vi "Patrycja_2.vi"() -> ()   [LabVIEW 2025]
uses:
  <vilib>/Instr/_visa.llb/VISA Flush IO Buffer Mask.ctl
  <vilib>/Utility/error.llb/Trim Whitespace One-Sided.vi
  <vilib>/Instr/_visa.llb/VISA Configure Serial Port (Instr).vi
panel:
  in  "Tab Control":T1(tab)
  out "Thermometer":dbl(slide) scale=0.0..100.0
  out "Temperatura wykres":dbl(graph)
  out "Temperatura liczba":dbl
  out "Temperatura max [C]":dbl
  out "Temperatura min[C]":dbl
  out "Temperatura średnia[C]":dbl
  out "Wilgotność wykres":dbl(graph)
  out "Tank":dbl(slide) scale=0.0..100.0
  out "wilgotność liczba":dbl
  out "Wilgotnosc max [%]":dbl
  out "Wilogtność min [%]":dbl
  out "Wilgotność średnia[%]":dbl
  out "Bardzo Suche":bool
  out "Punkt Rosy":dbl format="%#_4g"
  out "Indeks ciepła":dbl format="%#_4g"
  out "Suche":bool
  out "Komfort":bool
  out "Wilgotno":bool
  out "Bardzo Wilgotno":bool
  out "Komfort":bool
  out "Uwaga":bool
  out "Duża Ostrożność":bool
  out "Niebezpieczne":bool
  out "Ekstremalnie niebezpieczne":bool
  out "wyświetlanie danych":string
  out "Czy dziła whlie":i32
  out "numeric - start/stop":dbl
  in  "START/STOP":bool
  out "wyświetlanie danych 2":string
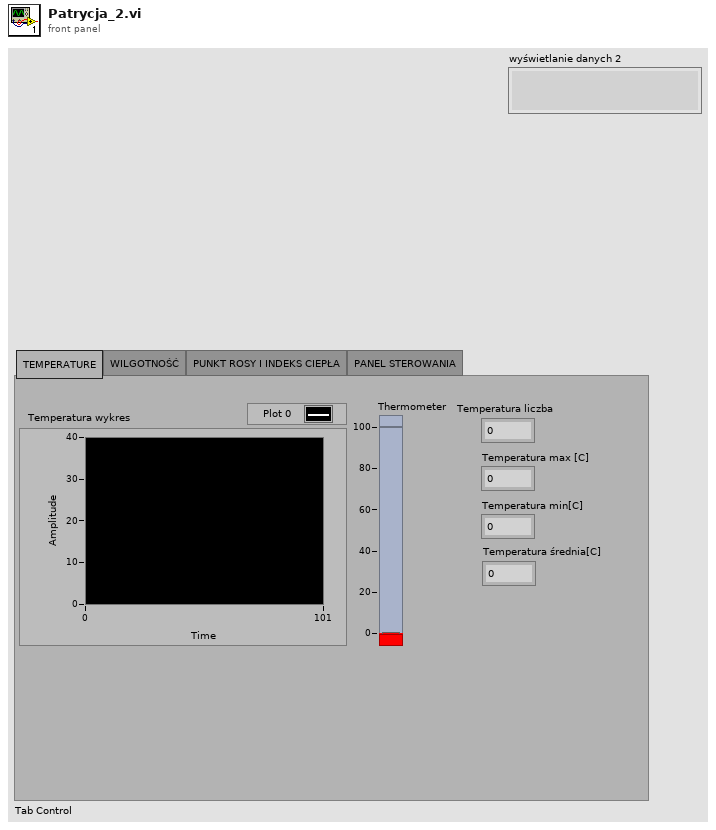
[diagram p1: front panel]
types:
  T1 = enum32{"TEMPERATURE", "WILGOTNOŚĆ", "PUNKT ROSY I INDEKS CIEPŁA", "PANEL STEROWANIA"}
  T2 = typedef "VISA Flush IO Buffer Mask.ctl" = u16
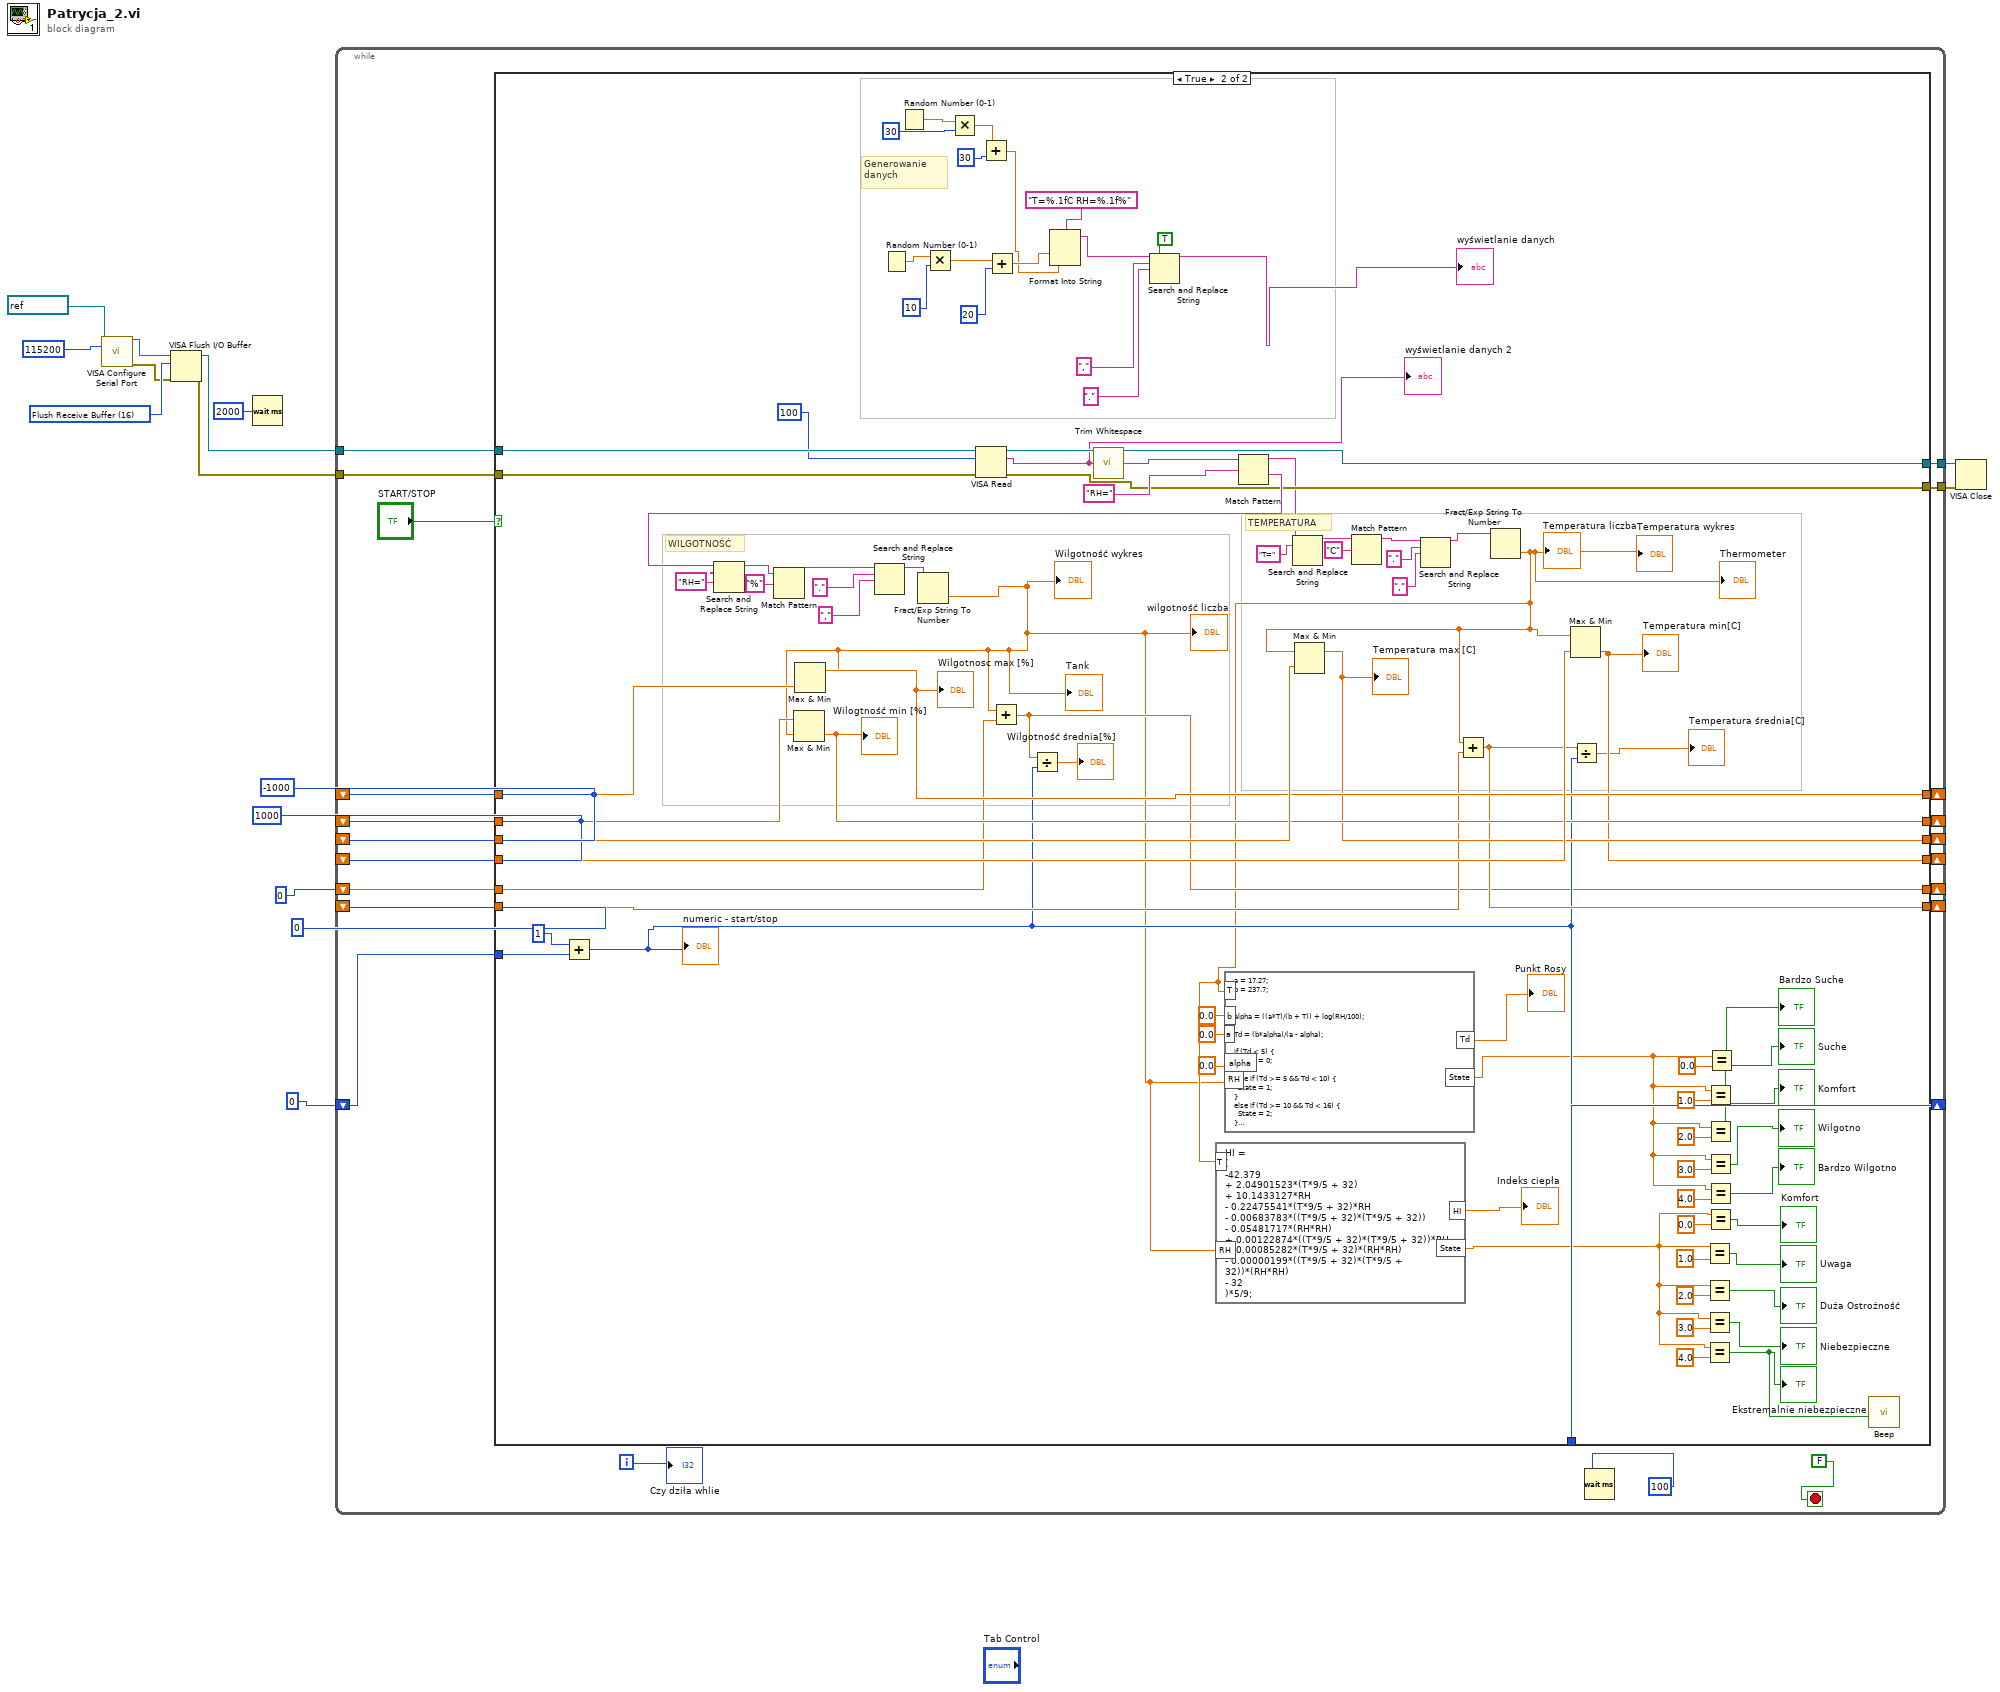
[diagram p0: block diagram]
diagram:
  w10 = T2 16 items=["Flush Receive Buffer"=16, "Write Transmit Buffer to Device"=32, "Flush Receive Buffer (No I/O)"=64, "Flush Transmit Buffer"=128] ("Mask")
  w14 = 1000
  w15 = -1000
  n1 = call-poly "VISA Configure Serial Port"("VISA resource name"=refnum<visa-resource-name> "COM7", "baud rate (9600)"=u32 115200) -> ("VISA resource name out"=w5:refnum<visa-resource-name>, "error out"=w4:errorcluster)  [unwired: 12 in]
  n2 = VISA Flush I/O Buffer(VISA resource name=w5, mask (16)=w10, error in (no error)=w4) -> (VISA resource name out=w8:refnum<visa-resource-name>, error out=w7:errorcluster)
  n3 = Wait (ms)(milliseconds to wait=u32 2000) -> ()  [unwired: 1 out]
  n4 = while {
    shift-right: [w32] -> _
    shift-left: w15 -> [w36]
    shift-right: [w31] -> _
    shift-left: w14 -> [w35]
    shift-right: [w30] -> _
    shift-left: w15 -> [w34]
    shift-right: [w29] -> _
    shift-left: w14 -> [w33]
    shift-right: [w25] -> _
    shift-left: 0 -> [w28]
    shift-right: [w26] -> _
    shift-left: 0 -> [w27]
    shift-right: [w21] -> _
    shift-left: 0 -> [w22]
    tunnel: [w19] -> w9
    tunnel: w8 -> [w18]
    tunnel: w7 -> [w17]
    tunnel: [w16] -> w6
    i -> [w24]
    stop <- FALSE stop-if-true
    n5 = case shown="True" "START/STOP" {
      tunnel: w36 -> [w45 w99]
      tunnel: w35 -> [w44 w98]
      tunnel: w34 -> [w43 w97]
      tunnel: w33 -> [w42 w96]
      tunnel: [w45 w95] -> w32
      tunnel: [w44 w94] -> w31
      tunnel: [w43 w93] -> w30
      tunnel: [w42 w92] -> w29
      tunnel: w28 -> [w41 w91]
      tunnel: w27 -> [w40 w90]
      tunnel: [w40 w89] -> w26
      tunnel: [w41 w77] -> w25
      tunnel: w22 -> [w46 w87]
      tunnel: [w46 w85] -> w21
      tunnel: [w38 w84] -> w19
      tunnel: w18 -> [w38 w80]
      tunnel: w17 -> [w39 w82]
      tunnel: [w39 w81] -> w16
      frame False {
      }
      frame True {
        # "Generowanie danych"
        # "WILGOTNOŚĆ"
        # "TEMPERATURA"
        n6 = Add(x=1, y=w87) -> (x+y=w85:i32)
        "numeric - start/stop" <- w85
        n7 = Random Number (0-1)() -> (number: 0 to 1=w112:dbl)
        n8 = Random Number (0-1)() -> (number: 0 to 1=w114:dbl)
        n9 = Multiply(x=w112, y=10) -> (x*y=w113:dbl)
        n10 = Multiply(x=w114, y=30) -> (x*y=w115:dbl)
        n11 = VISA Read(VISA resource name=w80, byte count=u32 100, error in (no error)=w82) -> (VISA resource name out=w84:refnum<visa-resource-name>, read buffer=w83:string, error out=w81:errorcluster)  [unwired: 1 out]
        "wyświetlanie danych 2" <- w83
        n12 = Add(x=w115, y=30) -> (x+y=w100:dbl)
        n13 = Add(x=w113, y=20) -> (x+y=w101:dbl)
        n14 = Format Into String(format string="T=%.1fC RH=%.1f%", w101, w100) -> (resulting string=w102:string)  [unwired: 2 in, 1 out]
        n15 = call <vilib>:"Trim Whitespace.vi"("string"=w83) -> ("trimmed string"=w125:string)  [unwired: 1 in]
        n16 = Search and Replace String(replace all?=TRUE, input string=w102, search string=",", replace string=".") -> (result string=→"wyświetlanie danych":string)  [unwired: 4 in, 3 out]
        n17 = Match Pattern(string=w125, regular expression="RH=") -> (before substring=w78:string, after substring=w129:string)  [unwired: 1 in, 2 out]
        n18 = Search and Replace String(input string=w129, search string="RH=") -> (result string=w130:string)  [unwired: 6 in, 3 out]
        n19 = Match Pattern(string=w130, regular expression="%") -> (before substring=w131:string)  [unwired: 1 in, 3 out]
        n20 = Search and Replace String(input string=w131, search string=".", replace string="," ("replace string (\"\")")) -> (result string=w132:string)  [unwired: 5 in, 3 out]
        n21 = Fract/Exp String To Number(string=w132) -> (number=w70:dbl)  [unwired: 3 in, 1 out]
        "Wilgotność wykres" <- w70
        "wilgotność liczba" <- w70
        "Tank" <- w70
        n22 = Max & Min(x=w98, y=w70) -> (min(x,y)=w94:dbl)  [unwired: 1 out]
        "Wilogtność min [%]" <- w94
        n23 = Max & Min(x=w70, y=w99) -> (max(x,y)=w95:dbl)  [unwired: 1 out]
        "Wilgotnosc max [%]" <- w95
        n24 = Add(x=w70, y=w91) -> (x+y=w77:dbl)
        n25 = Divide(x=w77, y=w85) -> (x/y=→"Wilgotność średnia[%]":dbl)
        n26 = Search and Replace String(input string=w78, search string="T=" ("replace string (\"\")")) -> (result string=w126:string)  [unwired: 6 in, 3 out]
        n27 = Match Pattern(string=w126, regular expression="C") -> (before substring=w127:string)  [unwired: 1 in, 3 out]
        n28 = Search and Replace String(input string=w127, search string=".", replace string="," ("replace string (\"\")")) -> (result string=w128:string)  [unwired: 5 in, 3 out]
        n29 = Fract/Exp String To Number(string=w128) -> (number=w71:dbl)  [unwired: 3 in, 1 out]
        "Temperatura wykres" <- w71
        "Temperatura liczba" <- w71
        "Thermometer" <- w71
        n30 = formula code="HI =\n(\n-42.379\n+ 2.04901523*(T*9/5 + 32)\n+ 10.1433127*RH\n- 0.22475541*(T*9/5 + 32)*RH\n- 0.00683783*((T*9/5 + 32)*(T*9/5 + 32))\n- 0.05481717*(RH*RH)\n+ 0.00122874*((T*9/5 + 32)*(T*9/5 + 32))*RH\n+ 0.00085282*(T*9/5 + 32)*(RH*RH)\n- 0.00000199*((T*9/5 + 32)*(T*9/5 + 32))*(RH*RH)\n- 32\n)*5/9;\n\n\nif (HI < 27) {\n  State = 0;\n}\nelse if (HI >= 27 && HI < 32) {\n  State = 1;\n}\nelse if (HI >= 32 && HI < 41) {\n  State = 2;\n}\nelse if (HI >= 41 && HI < 54) {\n  State = 3;\n}\nelse {\n  State = 4;\n}"("T"=w71, "RH"=w70) -> ("HI"=→"Indeks ciepła":dbl, "State"=w58:dbl)
        n31 = formula code="a = 17.27;\nb = 237.7;\n\n\nalpha = ((a*T)/(b + T)) + log(RH/100);\n\nTd = (b*alpha)/(a - alpha);\n\nif (Td < 5) {\n  State = 0;\n}\nelse if (Td >= 5 && Td < 10) {\n  State = 1;\n}\nelse if (Td >= 10 && Td < 16) {\n  State = 2;\n}\nelse if (Td >= 16 && Td < 20) {\n  State = 3;\n}\nelse {\n  State = 4;\n}"("T"=w71, "RH"=w70, "a"=0.0 ("input variable"), "b"=0.0 ("input variable"), "alpha"=0.0 ("input variable")) -> ("Td"=→"Punkt Rosy":dbl, "State"=w57:dbl)
        n32 = Max & Min(x=w71, y=w97) -> (max(x,y)=w93:dbl)  [unwired: 1 out]
        "Temperatura max [C]" <- w93
        n33 = Add(x=w71, y=w90) -> (x+y=w89:dbl)
        n34 = Max & Min(x=w71, y=w96) -> (min(x,y)=w92:dbl)  [unwired: 1 out]
        "Temperatura min[C]" <- w92
        n35 = Divide(x=w89, y=w85) -> (x/y=→"Temperatura średnia[C]":dbl)
        n36 = Equal?(x=w58, y=1.0) -> (x = y?=→"Uwaga":bool)
        n37 = Equal?(x=w58, y=2.0) -> (x = y?=→"Duża Ostrożność":bool)
        n38 = Equal?(x=w58, y=3.0) -> (x = y?=→"Niebezpieczne":bool)
        n39 = Equal?(x=w58, y=4.0) -> (x = y?=w47:bool)
        "Ekstremalnie niebezpieczne" <- w47
        n40 = Equal?(x=w57, y=1.0) -> (x = y?=→"Suche":bool)
        n41 = Equal?(x=w57, y=2.0) -> (x = y?=→"Komfort":bool)
        n42 = Equal?(x=w57, y=3.0) -> (x = y?=→"Wilgotno":bool)
        n43 = Equal?(x=w57, y=4.0) -> (x = y?=→"Bardzo Wilgotno":bool)
        n44 = Equal?(x=w58, y=0.0) -> (x = y?=→"Komfort":bool)
        n45 = Equal?(x=w57, y=0.0) -> (x = y?=→"Bardzo Suche":bool)
        n46 = call <vilib>:"Beep.vi"("use system alert? (T)"=w47) -> ()  [unwired: 11 in]
      }
    }
    n47 = Wait (ms)(milliseconds to wait=u32 100) -> ()  [unwired: 1 out]
    "Czy dziła whlie" <- w24
  }
  n48 = VISA Close(VISA resource name=w9, error in (no error)=w6) -> ()  [unwired: 1 out]
